vi "getvcan3setting.vi"(8 "error in (no error)":errorcluster, 11 "hObject":i32) -> (0 "error out":errorcluster, 2 "SVCAN3Setting":T1, 3 "hObject Out":i32)   [LabVIEW 2009]
doc: "this vi returns the SVCAN3Settings from the device\n\n12/21/2010 1.0.0 jyg\n- initial release"
uses:
  ctl svcansetting.ctl
  NEO VI Example/data/icsneo40.dll
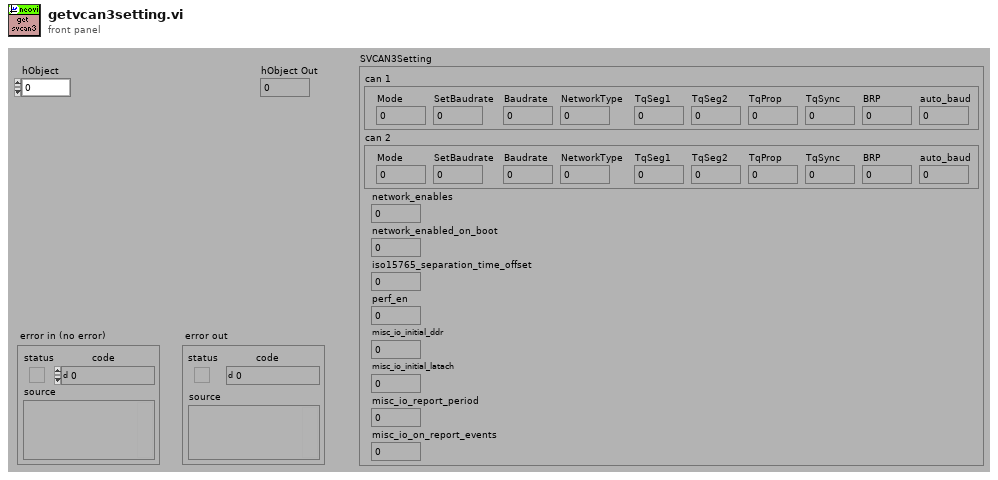
[diagram p1: front panel]
types:
  T1 = typedef "ctl SVCANSetting.ctl" = cluster{"can 1":cluster{"Mode":u8, "SetBaudrate":u8, "Baudrate":u8, "NetworkType":u8, "TqSeg1":u8, "TqSeg2":u8, "TqProp":u8, "TqSync":u8, "BRP":u16, "auto_baud":u16}, "can 2":cluster{"Mode":u8, "SetBaudrate":u8, "Baudrate":u8, "NetworkType":u8, "TqSeg1":u8, "TqSeg2":u8, "TqProp":u8, "TqSync":u8, "BRP":u16, "auto_baud":u16}, "network_enables":u16, "network_enabled_on_boot":u16, "iso15765_separation_time_offset":i16, "perf_en":u16, "misc_io_initial_ddr":u16, "misc_io_initial_latach":u16, "misc_io_report_period":u16, "misc_io_on_report_events":u16}
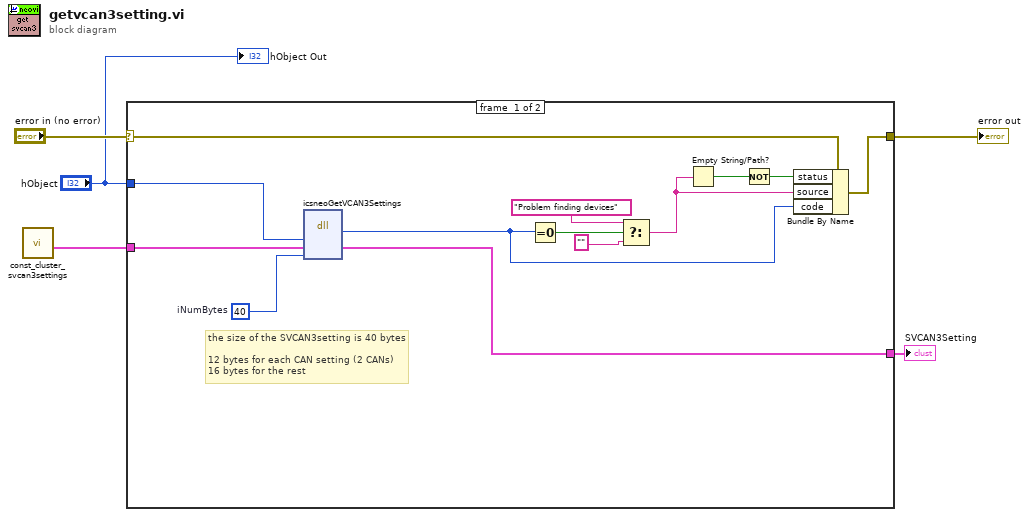
[diagram p0: block diagram]
diagram:
  n1 = call "const_cluster_svcan3settings.vi"() -> ("SVCAN3Settings"=w2:T1)
  n2 = case shown="No Error" "error in (no error)" {
    selector: "error in (no error)" -> [w14 w19]
    tunnel: "hObject" -> [w8 _]
    tunnel: [w15 w19] -> w5
    tunnel: w2 -> [w9 _]
    tunnel: [w7 _] -> w1
    frame #0 {
      w6 = 40  # iNumBytes
      # "the size of the SVCAN3setting is 40 bytes\n\n12 bytes for each CAN setting (2 CANs)\n16 bytes for the rest"
      n3 = dll-call lib="C:/WINDOWS/system32/icsneo40.dll" fn="icsneoGetVCAN3Settings"("hObject"=w8, "SVCAN3Setting"=w9, "iNumBytes"=w6) -> ("return type"=w13:i32, "SVCAN3Setting"=w7:T1)  [unwired: 5 in, 2 out]
      n4 = Equal To 0?(x=w13) -> (x = 0?=w12:bool)
      n5 = Select(t="Problem finding devices", s=w12, f="") -> (s? t:f=w11:string)
      n6 = Empty String/Path?(string/path=w11) -> (empty?=w17:bool)
      n7 = Not(x=w17) -> (.not. x?=w16:bool)
      n8 = Bundle By Name(cluster=w14, "status"=w16, "source"=w11, "code"=w13) -> (w15:errorcluster)
    }
    frame #1 {
    }
  }
  "error out" <- w5
  "SVCAN3Setting" <- w1
  "hObject Out" <- "hObject"
